vi "CAL time.vi"(7 "reference":refnum<vi>, 8 "error in (no error)":errorcluster, 9 "S2":dbl=12.0, 10 "S1":dbl=11.0, 11 "appended array":waveform(dbl)[](array[waveform])) -> (0 "error out":errorcluster, 3 "CAl VAlUE":T1)   [LabVIEW 2011]
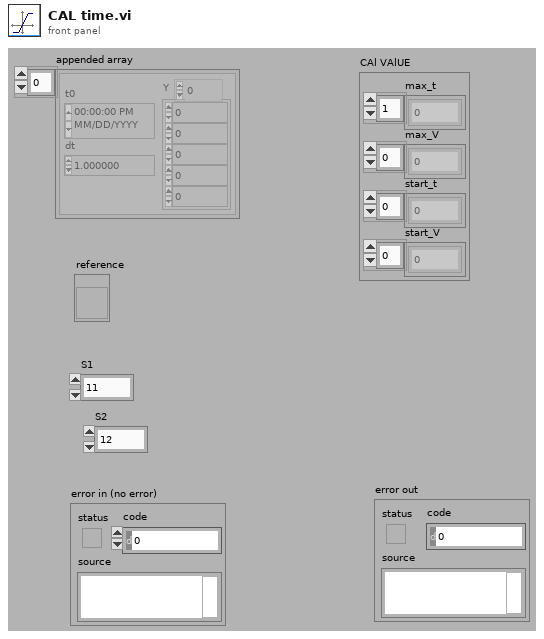
[diagram p1: front panel]
types:
  T1 = cluster{"max_t":dbl[], "max_V":dbl[], "start_t":dbl[], "start_V":dbl[]}
  T2 = cluster{"Width":u16, "Style":enum32{"Solid", "Dash", "Dot", "DashDot", "DashDotDot"}}
  T3 = typedef "LVRectTypeDef.ctl" = cluster{"left":i16, "top":i16, "right":i16, "bottom":i16}
  T4 = typedef "LVPoint32TypeDef.ctl" = cluster{"Horizontal":i32, "Vertical":i32}
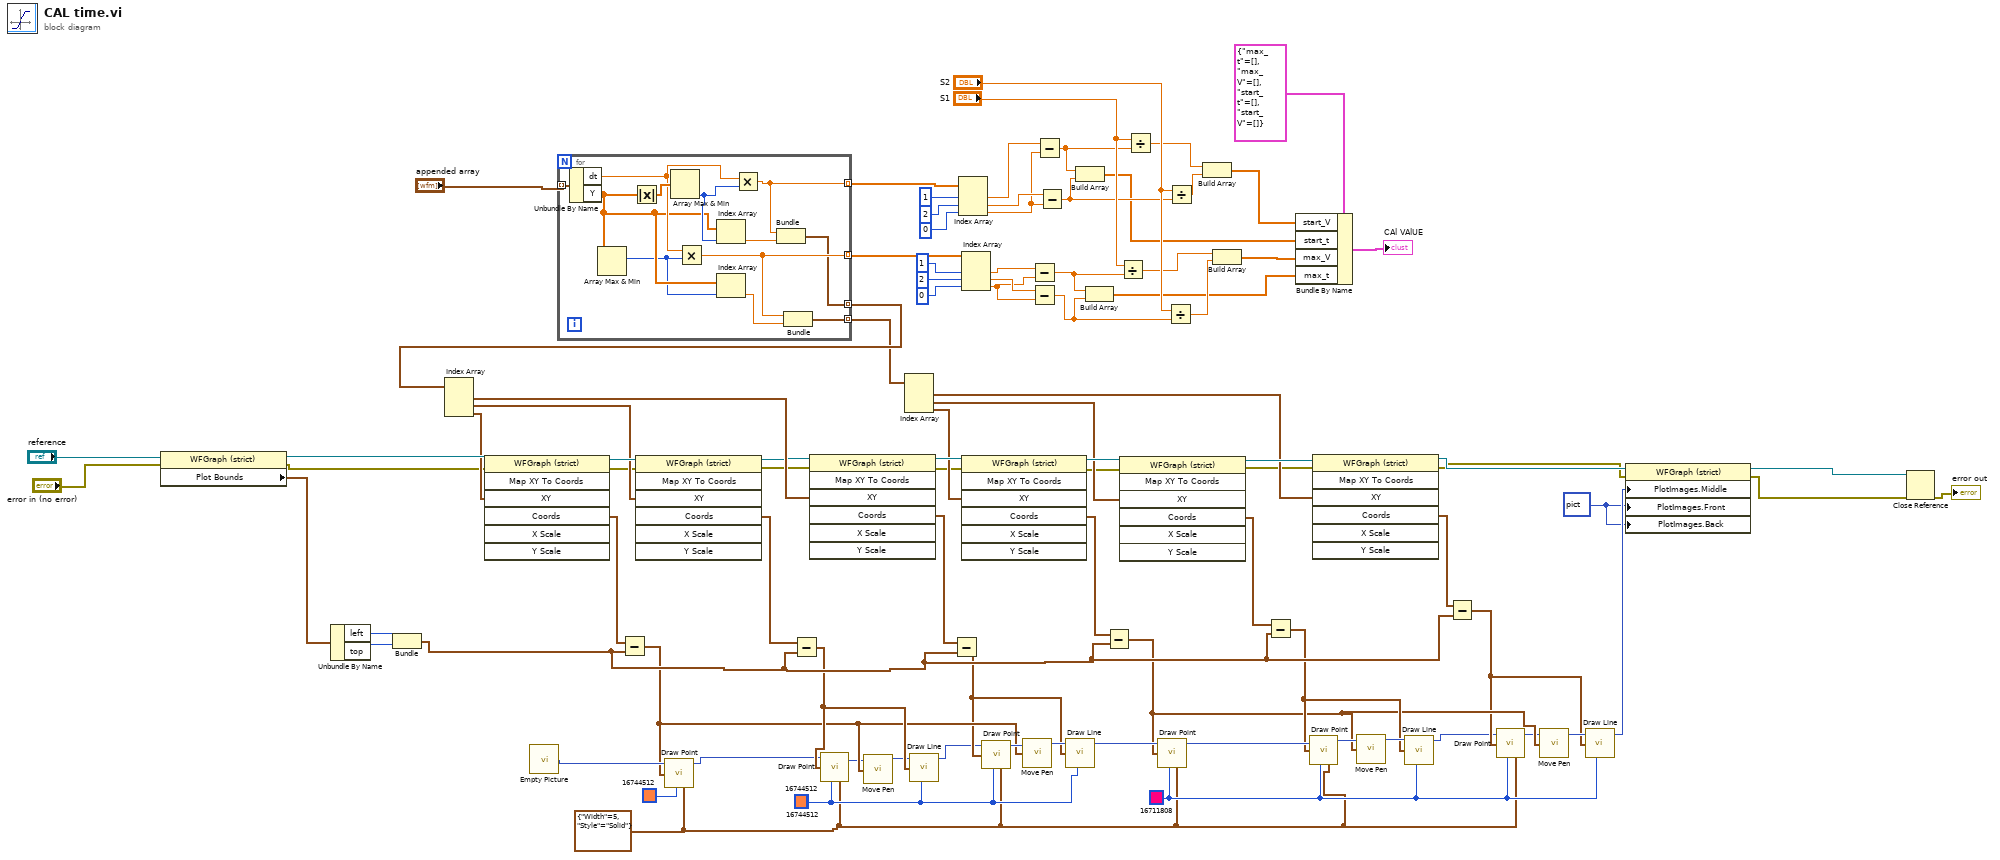
[diagram p0: block diagram]
diagram:
  w1 = picture data[5B] ("曲线图像:前景")
  w6 = u32 16711808 ("color(black)")
  (unwired) u32 16744512 ("color(black)")
  w7 = u32 16744512 ("color(black)")
  w5 = T2 {"Width"=5, "Style"=enum."Solid"} ("pen")
  n1 = property class="WFGraph (strict)"(reference="reference", error in="error in (no error)") -> (reference out=w55:refnum<vi>, error out=w9:errorcluster, "Plot Bounds"=w61:T3)
  n2 = Unbundle By Name(w61) -> ("left"=w60:i16, "top"=w59:i16)
  n3 = Bundle("left"=w60, "top"=w59) -> (w37:cluster{"left":i16, "top":i16})  [unwired: 1 out]
  n4 = call "Empty Picture"() -> ("empty picture"=w36:picture)
  n5 = for {
    tunnel: "appended array" -> [w106] mode=indexing
    tunnel: [w100] -> w65 mode=indexing
    tunnel: [w98] -> w90 mode=indexing
    tunnel: [w96] -> w58 mode=indexing
    tunnel: [w95] -> w57 mode=indexing
    n6 = Unbundle By Name(w106) -> ("dt"=w104:dbl, "Y"=w102:dbl[])
    n7 = Array Max & Min(array=w102) -> (max index (indices)=w101:i32)  [unwired: 3 out]
    n8 = Absolute Value(x=w102) -> (abs(x)=w105:dbl[])
    n9 = Array Max & Min(array=w105) -> (min index (indices)=w103:i32)  [unwired: 3 out]
    n10 = Multiply(x=w104, y=w101) -> (x*y=w98:dbl)
    n11 = Index Array(array=w102, index=w103) -> (element=w99:dbl)
    n12 = Index Array(array=w102, index=w101) -> (element=w97:dbl)
    n13 = Multiply(x=w104, y=w103) -> (x*y=w100:dbl)
    n14 = Bundle(w100, w99) -> (w96:cluster{dbl, dbl})  [unwired: 1 out]
    n15 = Bundle(w98, w97) -> (w95:cluster{dbl, dbl})  [unwired: 1 out]
  }
  n16 = Index Array(array=w58) -> (element #1=w56:cluster{dbl, dbl}, element #2=w47:cluster{dbl, dbl}, element #3=w48:cluster{dbl, dbl})  [unwired: 3 in]
  n17 = invoke class="WFGraph (strict)" method="Map XY To Coords"(reference=w55, error in=w9, "XY"=w48) -> (reference out=w54:refnum<vi>, error out=w10:errorcluster, "Coords"=w43:T4)  [unwired: 4 in, 4 out]
  n18 = Subtract(x=w43, y=w37) -> (x-y=w30:T4)
  n19 = invoke class="WFGraph (strict)" method="Map XY To Coords"(reference=w54, error in=w10, "XY"=w47) -> (reference out=w53:refnum<vi>, error out=w11:errorcluster, "Coords"=w42:T4)  [unwired: 4 in, 4 out]
  n20 = call <vilib>:"Draw Point.vi"("picture"=w36, "point(x,y)"=w30, "color(black)"=u32 16744512, "pen"=w5) -> ("new picture"=w25:picture)  [unwired: 5 out]
  n21 = Subtract(x=w42, y=w37) -> (x-y=w35:T4)
  n22 = invoke class="WFGraph (strict)" method="Map XY To Coords"(reference=w53, error in=w11, "XY"=w56) -> (reference out=w52:refnum<vi>, error out=w12:errorcluster, "Coords"=w41:T4)  [unwired: 4 in, 4 out]
  n23 = call <vilib>:"Draw Point.vi"("picture"=w25, "point(x,y)"=w35, "color(black)"=w7, "pen"=w5) -> ("new picture"=w26:picture)  [unwired: 5 out]
  n24 = call <vilib>:"Move Pen.vi"("new position"=w30, "picture"=w26) -> ("new picture"=w27:picture)  [unwired: 1 in, 2 out]
  n25 = Index Array(array=w57) -> (element #1=w44:cluster{dbl, dbl}, element #2=w45:cluster{dbl, dbl}, element #3=w46:cluster{dbl, dbl})  [unwired: 3 in]
  n26 = call <vilib>:"Draw Line.vi"("picture"=w27, "end point"=w35, "color(black)"=w7) -> ("new picture"=w28:picture)  [unwired: 2 in, 4 out]
  n27 = Subtract(x=w41, y=w37) -> (x-y=w29:T4)
  n28 = Index Array(array=w65, index #1=1 ("index"), index #2=2 ("index"), index #3=0 ("index")) -> (element #1=w87:dbl, element #2=w86:dbl, element #3=w85:dbl)
  n29 = Index Array(array=w90, index #1=1 ("index"), index #2=2 ("index"), index #3=0 ("index")) -> (element #1=w84:dbl, element #2=w83:dbl, element #3=w82:dbl)
  n30 = invoke class="WFGraph (strict)" method="Map XY To Coords"(reference=w52, error in=w12, "XY"=w46) -> (reference out=w51:refnum<vi>, error out=w13:errorcluster, "Coords"=w40:T4)  [unwired: 4 in, 4 out]
  n31 = call <vilib>:"Draw Point.vi"("picture"=w28, "point(x,y)"=w29, "color(black)"=w7, "pen"=w5) -> ("new picture"=w34:picture)  [unwired: 5 out]
  n32 = call <vilib>:"Move Pen.vi"("new position"=w30, "picture"=w34) -> ("new picture"=w33:picture)  [unwired: 1 in, 2 out]
  n33 = Subtract(x=w84, y=w82) -> (x-y=w76:dbl)
  n34 = Subtract(x=w83, y=w82) -> (x-y=w75:dbl)
  n35 = Subtract(x=w87, y=w85) -> (x-y=w78:dbl)
  n36 = Subtract(x=w86, y=w85) -> (x-y=w77:dbl)
  n37 = call <vilib>:"Draw Line.vi"("picture"=w33, "end point"=w29, "color(black)"=w7) -> ("new picture"=w24:picture)  [unwired: 2 in, 4 out]
  n38 = Build Array(w78, w77) -> (w69:dbl[])
  n39 = Build Array(w76, w75) -> (w67:dbl[])
  n40 = Subtract(x=w40, y=w37) -> (x-y=w20:T4)
  n41 = Divide(x="S1", y=w76) -> (x/y=w72:dbl)
  n42 = invoke class="WFGraph (strict)" method="Map XY To Coords"(reference=w51, error in=w13, "XY"=w45) -> (reference out=w50:refnum<vi>, error out=w14:errorcluster, "Coords"=w39:T4)  [unwired: 4 in, 4 out]
  n43 = Divide(x="S1", y=w78) -> (x/y=w74:dbl)
  n44 = call <vilib>:"Draw Point.vi"("picture"=w24, "point(x,y)"=w20, "color(black)"=w6, "pen"=w5) -> ("new picture"=w23:picture)  [unwired: 5 out]
  n45 = Divide(x="S2", y=w75) -> (x/y=w71:dbl)
  n46 = Divide(x="S2", y=w77) -> (x/y=w73:dbl)
  n47 = Build Array(w74, w73) -> (w70:dbl[])
  n48 = Build Array(w72, w71) -> (w68:dbl[])
  n49 = Subtract(x=w39, y=w37) -> (x-y=w21:T4)
  n50 = Bundle By Name(cluster=T1 {"max_t"=[], "max_V"=[], "start_t"=[], "start_V"=[]}, "start_V"=w70, "start_t"=w69, "max_V"=w68, "max_t"=w67) -> (→"CAl VAlUE":T1)
  n51 = call <vilib>:"Draw Point.vi"("picture"=w23, "point(x,y)"=w21, "color(black)"=w6, "pen"=w5) -> ("new picture"=w22:picture)  [unwired: 5 out]
  n52 = invoke class="WFGraph (strict)" method="Map XY To Coords"(reference=w50, error in=w14, "XY"=w44) -> (reference out=w49:refnum<vi>, error out=w16:errorcluster, "Coords"=w38:T4)  [unwired: 4 in, 4 out]
  n53 = call <vilib>:"Move Pen.vi"("new position"=w20, "picture"=w22) -> ("new picture"=w32:picture)  [unwired: 1 in, 2 out]
  n54 = call <vilib>:"Draw Line.vi"("picture"=w32, "end point"=w21, "color(black)"=w6) -> ("new picture"=w17:picture)  [unwired: 2 in, 4 out]
  n55 = Subtract(x=w38, y=w37) -> (x-y=w19:T4)
  n56 = call <vilib>:"Draw Point.vi"("picture"=w17, "point(x,y)"=w19, "color(black)"=w6, "pen"=w5) -> ("new picture"=w18:picture)  [unwired: 5 out]
  n57 = call <vilib>:"Move Pen.vi"("new position"=w20, "picture"=w18) -> ("new picture"=w31:picture)  [unwired: 1 in, 2 out]
  n58 = call <vilib>:"Draw Line.vi"("picture"=w31, "end point"=w19, "color(black)"=w6) -> ("new picture"=w15:picture)  [unwired: 2 in, 4 out]
  n59 = property class="WFGraph (strict)"(reference=w49, error in=w16, "PlotImages.Middle"=w15, "PlotImages.Front"=w1, "PlotImages.Back"=w1) -> (reference out=w64:refnum<vi>, error out=w63:errorcluster)
  n60 = Close Reference(reference=w64, error in (no error)=w63) -> (error out=→"error out":errorcluster)
